vi "Subvi FIFO OUT.vi"(6 "FIFO OUT debug":bool, 9 "Count":u32, 11 "FIFO OUT":refnum<k21>="FIFO OUT a") -> (2 "FIFO OUT free spots":u32)   [LabVIEW 2017]
uses:
  <vilib>/rvi/DataTransferAndStorage/Container/Common/niFpgaContainerExecOnDevCompGetState.vi
  <vilib>/rvi/Emulation/niFpgaEmulationIsFPGAContextNoSignature.vi
  <vilib>/rvi/Emulation/niFpgaSctlEmulationGetInTimedLoop.vi
  <vilib>/rvi/errors/niFpgaSetErrorForExecOnDevCompSimple.vi
  <vilib>/rvi/eio/common/nirviEmuReportErrorAndStop.vi
  <vilib>/rvi/DataTransferAndStorage/Container/Common/niFpgaContainerGetUniqueNameForEmu.vi
  <vilib>/rvi/FIFO/Fifo_Resource/nirvififoEmulationSetSize.vi
  <vilib>/rvi/FIFO/Fifo_Resource/nirviFifoEmulationQueueMgr.vi
  <instcachedir>/0/nirviFifoEmulationQueueMgr_E5CAEC123FF24DC58D834DCA3CDAA9B5.lvgen/nirviFifoEmulationQueueMgr_E5CAEC123FF24DC58D834DCA3CDAA9B5_001.vi
  <vilib>/rvi/FIFO/Fifo_Resource/nirvififoEmulationDetermineInputValidOut.vi
  <vilib>/rvi/FIFO/Fifo_Resource/nirvififoEmulationCreateLock.vi
  <vilib>/rvi/Emulation/niFpgaProcessEmulError.vi
  <vilib>/rvi/FIFO/Fifo_Resource/nirvififoEmulationObtainLock.vi
  <vilib>/rvi/FIFO/Fifo_Resource/nirvififoEmulationReleaseLock.vi
  <vilib>/rvi/occurrence/nirviWaitOnOccurrenceBase.vi
  <vilib>/rvi/errors/nirviReportUnexpectedCaseInternalError.vi
  <vilib>/rvi/errors/nirviReportUnexpectedCaseInternalError (U32).vi
  <vilib>/Utility/error.llb/Clear Errors.vi
  <vilib>/rvi/interface/RandomDataEmulation/niFpgaRandomDataHandleErrors.vi
  GV FIFO OUT gate.vi
  GV gated pixel clock change.vi
  <vilib>/rvi/DataTransferAndStorage/Container/XNode/niFpgaContainer.xnode
  <vilib>/rvi/FIFO/Fifo_Resource/niFpgaFifoEmulationRefIn.vi
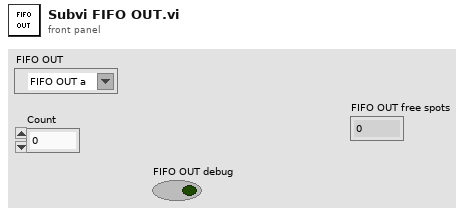
[diagram p1: front panel]
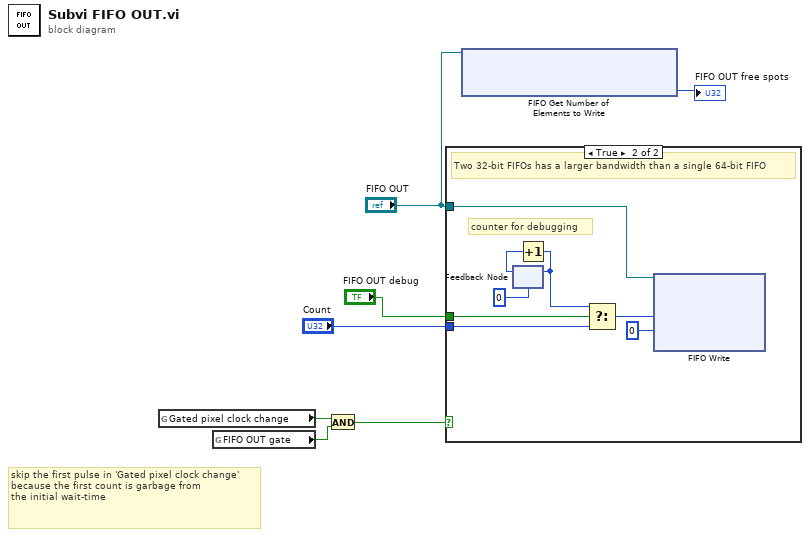
[diagram p0: block diagram]
diagram:
  # "skip the first pulse in 'Gated pixel clock change'\nbecause the first count is garbage from\nthe initial wait-time"
  n1 = global read "GV gated pixel clock change.vi" "Gated pixel clock change"() -> (w2:bool)
  n2 = global read "GV FIFO OUT gate.vi" "FIFO OUT gate"() -> (w7:bool)
  n3 = And(x=w2, y=w7) -> (x .and. y?=w1:bool)
  n4 = case shown="True" w1 {
    tunnel: "FIFO OUT debug" -> [_ w13]
    tunnel: "Count" -> [_ w12]
    tunnel: "FIFO OUT" -> [_ w10]
    frame False {
    }
    frame True {
      # "counter for debugging"
      # "Two 32-bit FIFOs has a larger bandwidth than a single 64-bit FIFO"
      n5 = feedback #1(u32 0) -> (w15:u32)
      n6 = Increment(x=w15) -> (x+1=w14:u32)
      n7 = feedback-in #1(w14) -> ()
      n8 = Select(t=w14, s=w13, f=w12) -> (s? t:f=w8:u32)
      n9 = xnode ("FIFO Write")("Element"=w8, "Timeout"=0, "FIFO In"=w10) -> ()  [unwired: 2 out]
    }
  }
  n10 = xnode ("FIFO Get Number of Elements to Write")("FIFO In"="FIFO OUT") -> ("Number of Elements to Write"=→"FIFO OUT free spots":u32)  [unwired: 1 out]
